vi "Actor Decorator.vi"(10 "Actor":refnum<class "Actor.lvclass">, 11 "Write Actor in":refnum<class "Actor Decorator.lvclass">) -> (3 "Write Actor out":refnum<class "Actor Decorator.lvclass">)   [LabVIEW 2021, in "AAM.lvlib" / "Actor Decorator.lvclass"]
uses:
  Actor Decorator.lvclass
  Actor/Actor.lvclass
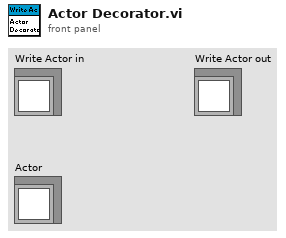
[diagram p1: front panel]
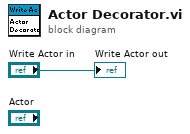
[diagram p0: block diagram]
diagram:
  "Write Actor out" <- "Write Actor in"
